vi "Set Mode.vi"(8 "error in":errorcluster, 10 "Mode":T1 items=["RUN"=6, "STANDBY"=7, "STOP"=8, "PAUSE"=9], 11 "CnPt in":refnum<class "CnPt.lvclass">) -> (0 "error out":errorcluster, 3 "CnPt out":refnum<class "CnPt.lvclass">)   [LabVIEW 2015, in "CnPt.lvclass"]
uses:
  CnPt.lvclass
  Mode.ctl
  <vilib>/MSR Consulting, LLC/General Reuse/Session APIs/Serial/Serial Session.lvclass
  CnPt.lvclass/CnPt.ctl
  <vilib>/MSR Consulting, LLC/General Reuse/Session APIs/Serial/Public/Asynchronous Write.vi
  <vilib>/MSR Consulting, LLC/General Reuse/Session APIs/Serial/Public/Asynchronous Read.vi
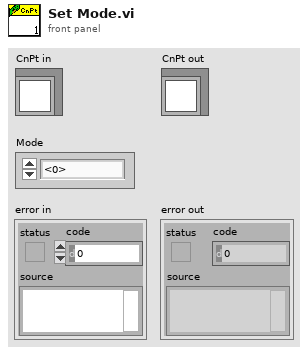
[diagram p1: front panel]
types:
  T1 = typedef "CnPt.lvclass/Mode.ctl" = u16
  T2 = typedef "Serial Session.lvclass/Session Handle.ctl" = refnum<data-value>
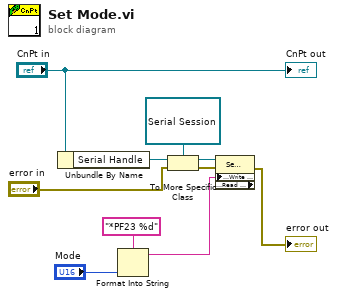
[diagram p0: block diagram]
diagram:
  n1 = Unbundle By Name("CnPt in") -> ("Serial Handle"=w10:T2)
  n2 = Format Into String(format string="*PF23 %d", "Mode") -> (resulting string=w1:string)  [unwired: 2 in, 1 out]
  n3 = To More Specific Class(target class=refnum<data-value> refnum, reference=w10, error in="error in") -> (specific class reference=w8:refnum<data-value>, error out=w7:errorcluster)
  n4 = property class="Serial Session" props=["Public:Write - Asynchronous", "Public:Read - Asynchronous"](reference=w8, error in=w7, "Public:Write - Asynchronous"=w1) -> (error out=→"error out":errorcluster)  [unwired: 2 out]
  "CnPt out" <- "CnPt in"
